vi "ULx Create Channel (CompI-Digital Input).vi"(0 "task in":refnum<k24>, 5 "ports":refnum<k21>, 11 "error in":errorcluster) -> (4 "task out":refnum<k24>, 15 "error out":errorcluster)   [LabVIEW 2020]
doc: "Creates channel(s) to measure digital signals. You cannot separate the ports into multiple channels."
uses:
  C:/Users/William/Documents/LV 2020 builds/LeaktestDAQ/Source-v33/ULx_LV.dll
  ULx_LV.dll
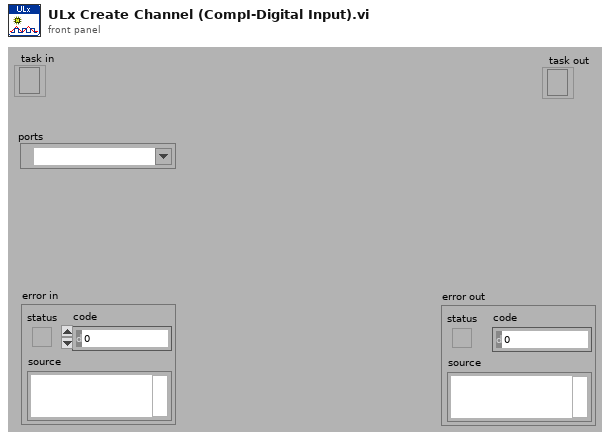
[diagram p1: front panel]
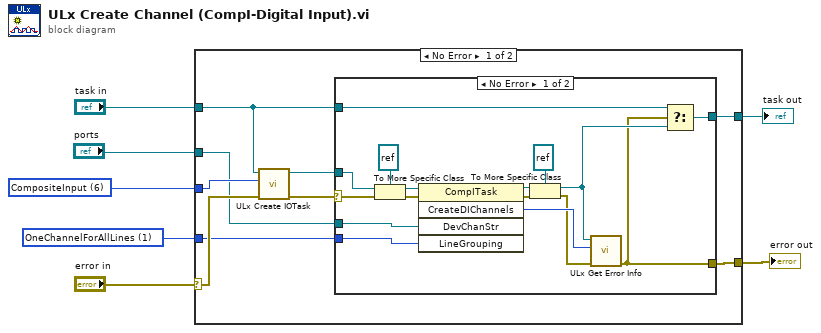
[diagram p0: block diagram]
diagram:
  w3 = 1 items=["OneChannelForAllLines"=1] ("line grouping")
  w2 = 6 items=["AnalogInput", "AnalogOutput", "DigitalInput", "DigitalOutput", "CounterInput", "CounterOutput", "CompositeInput", "CompositeOutput", "TemperatureInput"] ("taskType")
  n1 = case shown="No Error" "error in" {
    selector: "error in" -> [w16 w36]
    tunnel: "task in" -> [w8 w35]
    tunnel: "ports" -> [w10 _]
    tunnel: w2 -> [w11 _]
    tunnel: [w14 w35] -> w5
    tunnel: [w13 w36] -> w4
    tunnel: w3 -> [w9 _]
    frame No Error {
      n2 = call "ULx Create IOTask.vi"("error in"=w16, "taskType"=w11, "i/o task in"=w8) -> ("error out"=w15:errorcluster, "i/o task out"=w12:refnum<k24>)  [unwired: 7 in]
      n3 = case shown="No Error" w15 {
        selector: w15 -> [w30 w34]
        tunnel: [w17 w34] -> w13
        tunnel: [w21 w33] -> w14
        tunnel: w12 -> [w28 _]
        tunnel: w10 -> [w27 _]
        tunnel: w9 -> [w25 _]
        tunnel: w8 -> [w19 w33]
        frame No Error {
          n4 = To More Specific Class(target class=refnum<k24> refnum, reference=w28, error in=w30) -> (specific class reference=w31:refnum<k24>, error out=w29:errorcluster)
          n5 = invoke class="CompITask" method="CreateDIChannels"(reference=w31, error in=w29, "DevChanStr"=w27, "LineGrouping"=w25) -> (reference out=w23:refnum<k24>, error out=w22:errorcluster, "CreateDIChannels"=w26:i32)  [unwired: 1 in, 2 out]
          n6 = To More Specific Class(target class=refnum<k24> refnum, reference=w23, error in=w22) -> (specific class reference=w20:refnum<k24>, error out=w18:errorcluster)
          n7 = call "ULx Get Error Info.vi"("error in"=w18, "ErrorCode"=w26, "task in"=w20) -> ("error out"=w17:errorcluster)  [unwired: 8 in]
          n8 = Select(t=w19, s=w17, f=w20) -> (s? t:f=w21:refnum<k24>)
        }
        frame Error {
        }
      }
    }
    frame Error {
    }
  }
  "error out" <- w4
  "task out" <- w5
